vi "Static_Drive_Config_names.vi"() -> (0 "Ch names":string[](array[string])=["Correction:Gain %:(CG)", "Dead:Band:(DB)", "Dead Band:Window:(DW)", "Encoder:Resolution:(ER)", "Step:Mode:(FSB)", "Position:Maintenance:(FSC)", "Stop on:Stall:(FSD)", "Activate OP1:on stall:(FSE)", "Stop on:Trigger 3:(FSF)", "OP2 in:Deadband:(FSG)", "Stall:Detect:(FSH)", "Limit:Disable:(LD)", "Motor:Resolution:(MR)", "Limit Switch:Sense:(OSA)", "Home:Position:(OSB)", "Home Switch:Sense:(OSC)", "Encoder Z:for Home:(OSD)", "Reference edge:of Home:(OSH)", "RS232 Echo:Control:(SSA)", "Buffer at:Limit:(SSG)", "Buffer at:Stop:(SSH)", "Indexer:Mode:(FSA)", "Type:For Example:ParkerX"])   [LabVIEW 2010]
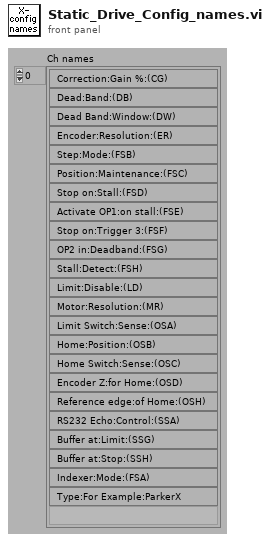
[diagram p1: front panel]
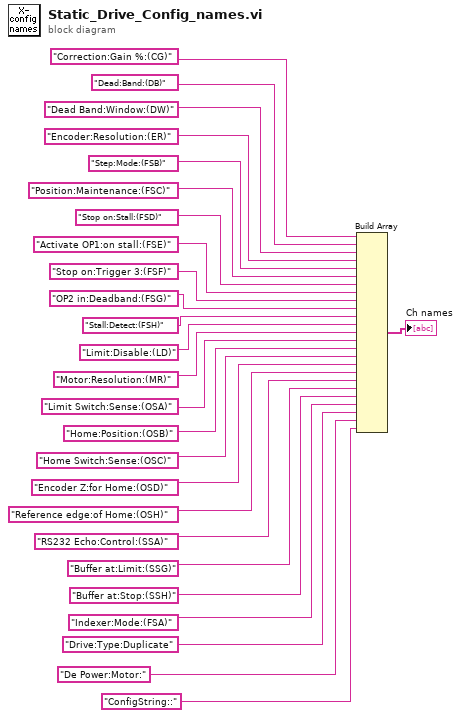
[diagram p0: block diagram]
diagram:
  n1 = Build Array("Correction:Gain %:(CG)", "Dead:Band:(DB)", "Dead Band:Window:(DW)", "Encoder:Resolution:(ER)", "Step:Mode:(FSB)", "Position:Maintenance:(FSC)", "Stop on:Stall:(FSD)", "Activate OP1:on stall:(FSE)", "Stop on:Trigger 3:(FSF)", "OP2 in:Deadband:(FSG)", "Stall:Detect:(FSH)", "Limit:Disable:(LD)", "Motor:Resolution:(MR)", "Limit Switch:Sense:(OSA)", "Home:Position:(OSB)", "Home Switch:Sense:(OSC)", "Encoder Z:for Home:(OSD)", "Reference edge:of Home:(OSH)", "RS232 Echo:Control:(SSA)", "Buffer at:Limit:(SSG)", "Buffer at:Stop:(SSH)", "Indexer:Mode:(FSA)", "Drive:Type:Duplicate", "De Power:Motor:", "ConfigString::") -> (→"Ch names":string[])
